vi "Q -- range -- gate  - not above.vi"(2 "gate":T1=enum."above", 3 "new state":T1=enum."above") -> (0 "new state out":T1)   [LabVIEW 2010]
uses:
  comparison control.ctl
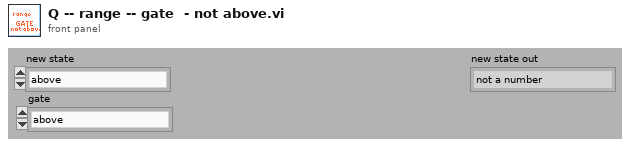
[diagram p1: front panel]
types:
  T1 = typedef "comparison control.ctl" = enum16{"not a number", "above", "in range", "below"}
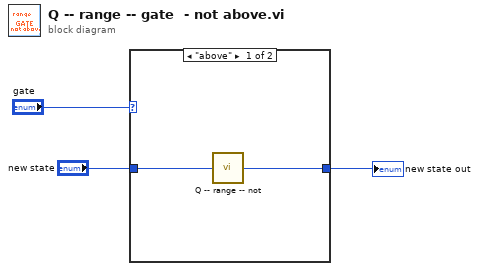
[diagram p0: block diagram]
diagram:
  n1 = case shown="\"above\"" "gate" {
    tunnel: [w4 w6] -> w3
    tunnel: "new state" -> [w5 w6]
    frame "above" {
      n2 = call "Q -- range -- not.vi"("new state"=w5) -> ("new state out"=w4:T1)
    }
    frame "below", Default {
    }
  }
  "new state out" <- w3
